vi "ping new test 001.vi"() -> ()   [LabVIEW 2019]
uses:
  <vilib>/Platform/TimedLoop/XDataNode/timing_clust.ctl
  <vilib>/Platform/TimedLoop/XDataNode/nitl_modes.ctl
  <vilib>/Platform/TimedLoop/XDataNode/wakeup.ctl
  <vilib>/platform/TimedLoop/XDataNode/XDataNode.xnode
  <vilib>/Platform/TimedLoop/XDataNode/XDNodeRunTimeDep.lvlib
panel:
  out "Waveform Chart":dbl(graph)
  in  "Stop":bool
  in  "error in":errorcluster
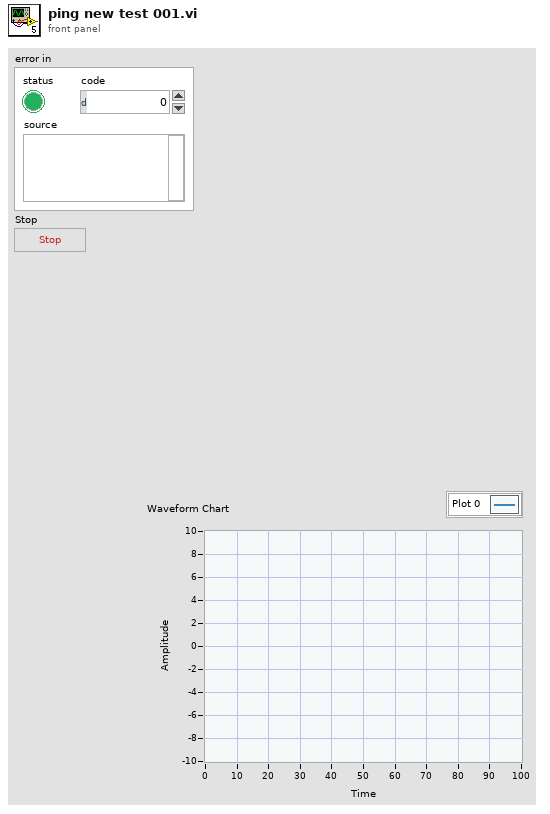
[diagram p1: front panel]
types:
  T1 = typedef "XDNodeRunTimeDep.lvlib/timing_clust.ctl" = cluster{"Expected End [f-1]":u64, "Actual End [f-1]":u64, "Finished Late? [f-1]":bool, "Expected End [i-1]":u64, "Actual End [i-1]":u64, "Finished Late? [i-1]":bool, "Expected Start [i]":u64, "Actual Start [i]":u64, "Expected Start [f]":u64, "Actual Start [f]":u64, "Source Name":string, "Structure Name":string, "Period":i64, "Deadline":i64, "Offset":i64, "Start":i64, "Priority":i32, "Timeout":i32, "Mode":T2, "Wakeup Reason":T3, "Error":errorcluster, "Source Type":string, "Secondary Source Type":string, "Global End Time":u64, "Global Start Time":u64, "Frame Duration":u64, "Iteration Duration":u64, "Assigned CPU":i32, "I/O Scan Engine Mode":u32}
  T2 = typedef "XDNodeRunTimeDep.lvlib/nitl_modes.ctl" = enum32{"No Change", "Process missed periods, maintain original phase", "Discard missed periods, maintain original phase", "Process missed periods, ignore original phase", "Discard missed periods, ignore original phase"}
  T3 = typedef "XDNodeRunTimeDep.lvlib/wakeup.ctl" = enum32{"Normal", "Aborted", "Asynchronous wakeup", "Timing source error", "Timed loop error", "Timeout"}
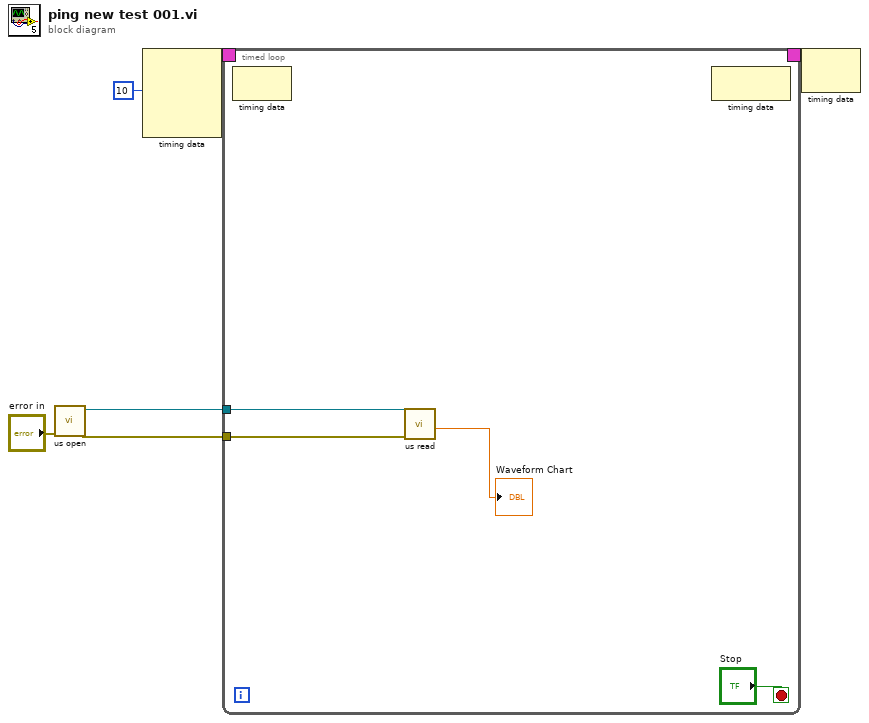
[diagram p0: block diagram]
diagram:
  n1 = call "us open.vi"("error in"="error in") -> ("error out"=w4:errorcluster, "output cluster"=w3:refnum<class "US sensor.lvclass">)  [unwired: 9 in]
  n2 = node-c288(i64 10 ("Period")) -> (w6:T1)  [unwired: 3 in]
  n3 = timed-loop {
    timing: w6 -> [_]
    timing-out: [_] -> w5
    tunnel: w4 -> [w10]
    tunnel: w3 -> [w9]
    stop <- "Stop" stop-if-true
    n4 = node-c288() -> ()  [unwired: 1 in, 1 out]
    n5 = call "us read.vi"("Error In"=w10, "my FPGA lib.lvlib:US sensor.lvclass"=w9) -> ("DC estimate (V)"=→"Waveform Chart":dbl)  [unwired: 6 in, 3 out]
    n6 = node-c288() -> ()  [unwired: 1 in, 1 out]
  }
  n7 = node-c288(w5) -> ()  [unwired: 1 out]
